vi "_getStartingIndex.vi"(10 "Starting Index In":u32[](array[numeric]), 11 "Waveforms":waveform(dbl)[](array[waveform])) -> (3 "Starting Index":u32[](array[numeric]))   [LabVIEW 2019]
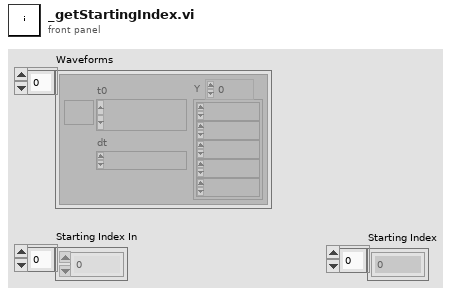
[diagram p1: front panel]
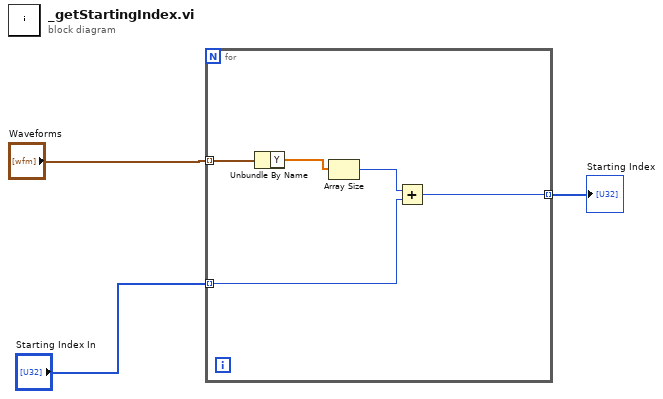
[diagram p0: block diagram]
diagram:
  n1 = for {
    tunnel: "Waveforms" -> [w8] mode=indexing
    tunnel: "Starting Index In" -> [w6] mode=indexing
    tunnel: [w4] -> w1 mode=indexing
    n2 = Unbundle By Name(w8) -> ("Y"=w7:dbl[])
    n3 = Array Size(array=w7) -> (size(s)=w5:i32)
    n4 = Add(x=w5, y=w6) -> (x+y=w4:u32)
  }
  "Starting Index" <- w1
